vi "Polymorphic Add.vi"() -> ()   [LabVIEW 2012]
panel:
  out "数组":i32[](array[numeric])
  out "数组":i32[](array[numeric])
  out "标量":i32
  out "数组":i32[](array[numeric])
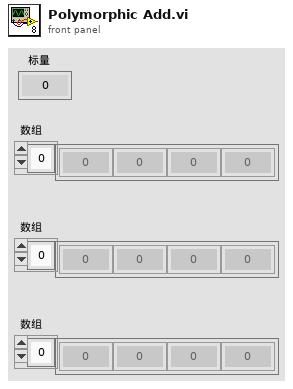
[diagram p1: front panel]
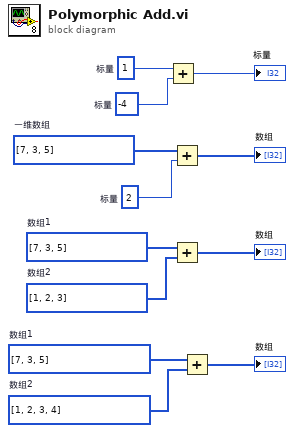
[diagram p0: block diagram]
diagram:
  w2 = i32[] [1, 2, 3, 4]  # 数组2
  w3 = i32[] [7, 3, 5]  # 数组1
  w7 = i32[] [1, 2, 3]  # 数组2
  w6 = i32[] [7, 3, 5]  # 数组1
  w12 = 1  # 标量
  w9 = i32[] [7, 3, 5]  # 一维数组
  w8 = 2  # 标量
  w11 = -4  # 标量
  n1 = Add ("加")(x=w12, y=w11) -> (x+y=→"标量":i32)
  n2 = Add ("加")(x=w9, y=w8) -> (x+y=→"数组":i32[])
  n3 = Add ("加")(x=w6, y=w7) -> (x+y=→"数组":i32[])
  n4 = Add ("加")(x=w3, y=w2) -> (x+y=→"数组":i32[])
